vi "OlympusInitialize.vi"(8 "error in (no error)":errorcluster, 11 "IX81 in":refnum<visa-resource-name>) -> (0 "error out":errorcluster, 2 "Focus Position":dbl, 3 "Prism Position (0: Bi)":enum16{"Bi", "Side"}(ring), 5 "Intensity [%]":dbl)   [LabVIEW 2018, in "Olympus IX BX Series.lvlib"]
uses:
  Olympus IX BX Series.lvlib
panel:
  out "IX81Objective":u16(ring) caption="Objective" items=["x 4", "x 10", "x 20", "x 40", "x 100"]
  out "IX81Filter":u16(ring)=6 caption="Filter:" items=["UV ", "CFP", "YFP", "RFP", "Cy5", "GFP", "BF"]
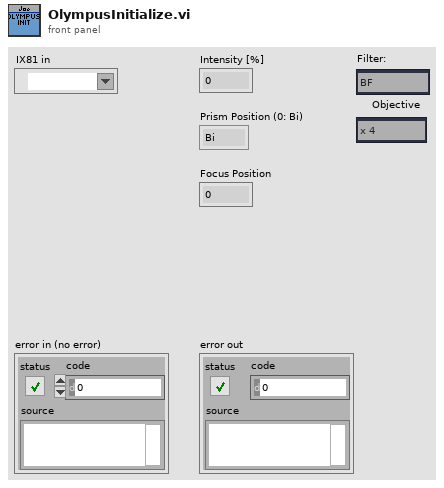
[diagram p1: front panel]
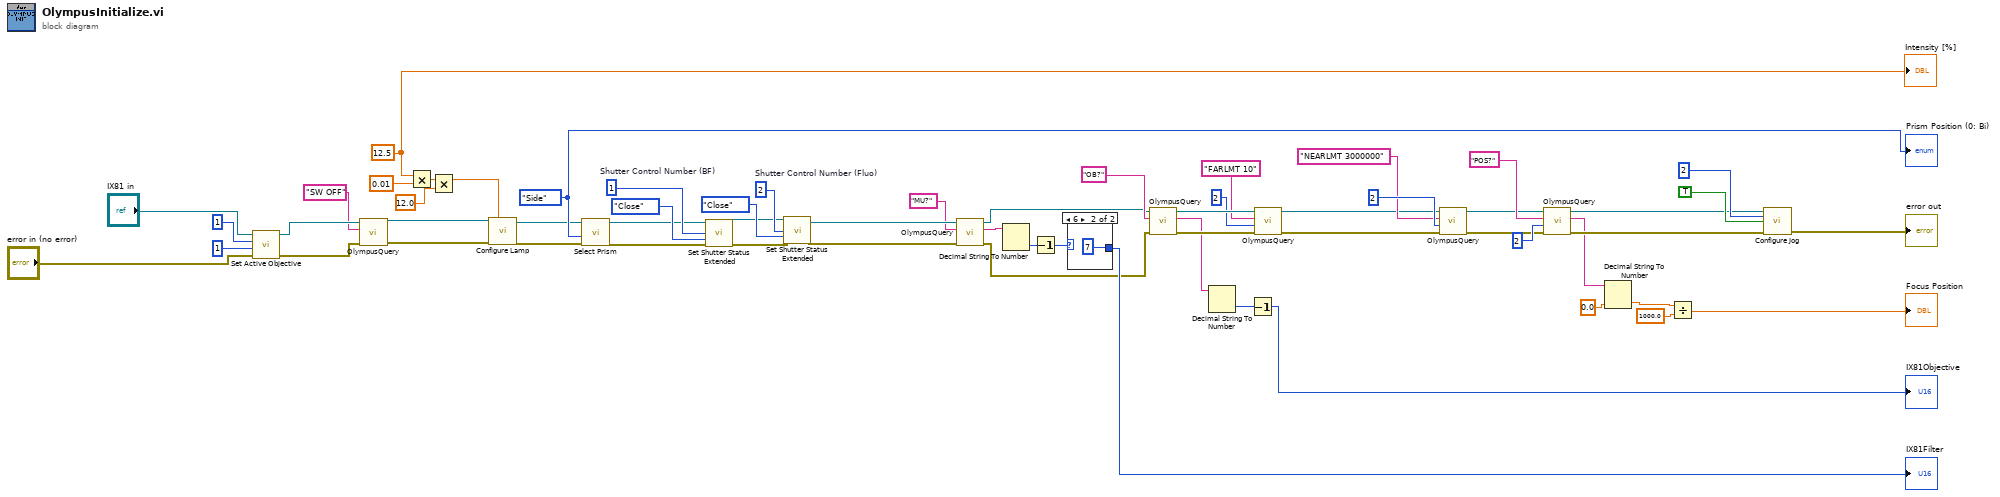
[diagram p0: block diagram]
diagram:
  w55 = 2  # Shutter Control Number (Fluo)
  w53 = 1  # Shutter Control Number (BF)
  w48 = enum16{"Bi", "Side"}."Side" ("Prism Position (0: Bi)")
  w39 = 12.5 ("Intensity [%]")
  n1 = call "Set Active Objective.vi"("error in (no error)"="error in (no error)", "Objective Number (1)"=1, "Device Number (1)"=1, "VISA Resource Name"="IX81 in") -> ("error out"=w33:errorcluster, "VISA Resource Name Out"=w32:refnum<visa-resource-name>)  [unwired: 6 in]
  n2 = call "OlympusQuery.vi"("error in (no error)"=w33, "String"="SW OFF", "VISA Resource Name In"=w32) -> ("error out"=w45:errorcluster, "VISA Resource Name Out"=w44:refnum<visa-resource-name>)  [unwired: 6 in, 1 out]
  n3 = Multiply(x=w39, y=0.01) -> (x*y=w40:dbl)
  n4 = Multiply(x=w40, y=12.0) -> (x*y=w42:dbl)
  n5 = call "Configure Lamp.vi"("VISA Resource Name"=w44, "Lamp Intensity (1.0 V)"=w42, "error in (no error)"=w45) -> ("VISA Resource Name Out"=w46:refnum<visa-resource-name>, "error out"=w47:errorcluster)  [unwired: 11 in]
  n6 = call "Select Prism.vi"("error in (no error)"=w47, "Prism Position (0: Bi)"=w48, "VISA Resource Name"=w46) -> ("error out"=w50:errorcluster, "VISA Resource Name Out"=w49:refnum<visa-resource-name>)  [unwired: 7 in]
  n7 = call "Set Shutter Status Extended.vi"("VISA Resource Name"=w49, "Shutter Control Number (1)"=w53, "Shutter Status (0: Open)"=enum16{"Open", "Close"}."Close", "error in (no error)"=w50) -> ("VISA Resource Name Out"=w52:refnum<visa-resource-name>, "error out"=w51:errorcluster)  [unwired: 10 in]
  n8 = call "Set Shutter Status Extended.vi"("VISA Resource Name"=w52, "Shutter Control Number (1)"=w55, "Shutter Status (0: Open)"=enum16{"Open", "Close"}."Close", "error in (no error)"=w51) -> ("VISA Resource Name Out"=w57:refnum<visa-resource-name>, "error out"=w58:errorcluster)  [unwired: 10 in]
  n9 = call "OlympusQuery.vi"("error in (no error)"=w58, "String"="MU?", "VISA Resource Name In"=w57) -> ("error out"=w1:errorcluster, "Result"=w18:string, "VISA Resource Name Out"=w2:refnum<visa-resource-name>)  [unwired: 6 in]
  n10 = Decimal String To Number(string=w18) -> (number=w19:i32)  [unwired: 2 in, 1 out]
  n11 = Decrement(x=w19) -> (x-1=w5:i32)
  n12 = case shown="6" w5 {
    selector: w5 -> [w61 _]
    tunnel: [w61 7] -> w4
    frame 0, Default {
    }
    frame 6 {
    }
  }
  "IX81Filter" <- w4
  n13 = call "OlympusQuery.vi"("error in (no error)"=w1, "String"="OB?", "VISA Resource Name In"=w2) -> ("error out"=w59:errorcluster, "Result"=w20:string, "VISA Resource Name Out"=w60:refnum<visa-resource-name>)  [unwired: 6 in]
  n14 = Decimal String To Number(string=w20) -> (number=w21:i32)  [unwired: 2 in, 1 out]
  n15 = Decrement(x=w21) -> (x-1=→"IX81Objective":i32)
  n16 = call "OlympusQuery.vi"("error in (no error)"=w59, "Device Number\n(1: -Condensor\n     - Objective\n     - Lamp\n     - Shutter\n2: - Z-Motion\n   - Autofocus)"=2 ("Device Number\n(1: -Condensor\n     - Objective\n     - Lamp\n     - Shutter\n2: - Z-Motion\n   - Autofocus)"), "String"="FARLMT 10", "VISA Resource Name In"=w60) -> ("error out"=w13:errorcluster, "VISA Resource Name Out"=w12:refnum<visa-resource-name>)  [unwired: 5 in, 1 out]
  n17 = call "OlympusQuery.vi"("error in (no error)"=w13, "Device Number\n(1: -Condensor\n     - Objective\n     - Lamp\n     - Shutter\n2: - Z-Motion\n   - Autofocus)"=2 ("Device Number\n(1: -Condensor\n     - Objective\n     - Lamp\n     - Shutter\n2: - Z-Motion\n   - Autofocus)"), "String"="NEARLMT 3000000", "VISA Resource Name In"=w12) -> ("error out"=w16:errorcluster, "VISA Resource Name Out"=w15:refnum<visa-resource-name>)  [unwired: 5 in, 1 out]
  n18 = call "OlympusQuery.vi"("error in (no error)"=w16, "Device Number\n(1: -Condensor\n     - Objective\n     - Lamp\n     - Shutter\n2: - Z-Motion\n   - Autofocus)"=2 ("Device Number\n(1: -Condensor\n     - Objective\n     - Lamp\n     - Shutter\n2: - Z-Motion\n   - Autofocus)"), "String"="POS?", "VISA Resource Name In"=w15) -> ("error out"=w27:errorcluster, "Result"=w26:string, "VISA Resource Name Out"=w28:refnum<visa-resource-name>)  [unwired: 5 in]
  n19 = Decimal String To Number(string=w26, default (0L)=0.0 ("default (0 I32)")) -> (number=w37:dbl)  [unwired: 1 in, 1 out]
  n20 = Divide(x=w37, y=1000.0) -> (x/y=→"Focus Position":dbl)
  n21 = call "Configure Jog.vi"("VISA Resource Name"=w28, "Device Number (1)"=2, "Enabled (False)"=TRUE, "error in (no error)"=w27) -> ("error out"=→"error out":errorcluster)  [unwired: 10 in, 1 out]
  "Prism Position (0: Bi)" <- w48
  "Intensity [%]" <- w39
